vi "sensor_lights_led.vi"() -> ()   [LabVIEW 2011]
panel:
  in  "stop":bool
  in  "y":dbl
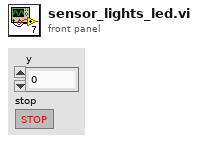
[diagram p1: front panel]
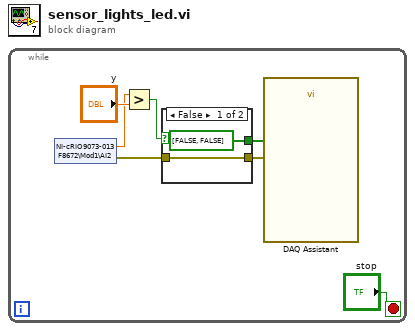
[diagram p0: block diagram]
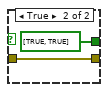
[diagram p2: hidden frame]
diagram:
  n1 = while {
    stop <- "stop" stop-if-true
    n2 = shared-variable "NI-cRIO9073-013F8672\\Mod1\\AI2"() -> (w5:dbl, error out=w4:errorcluster)  [unwired: 1 in]
    n3 = Greater?(x=w5, y="y") -> (0:w7:bool)
    n4 = case shown="False" w7 {
      tunnel: w4 -> [w8 w10]
      tunnel: [bool[] [FALSE, FALSE] ("data") bool[] [TRUE, TRUE] ("data")] -> w2
      tunnel: [w8 w10] -> w1
      frame False {
      }
      frame True {
      }
    }
    n5 = call "DAQ Assistant"("data"=w2, "error in"=w1) -> ()  [unwired: 16 in, 2 out]
  }
